vi "Timestamp_with_milliseconds.vi"(0 "Input Time":string="07:54:55.584 08/08/18") -> (4 "Output Time":string)   [LabVIEW 2014]
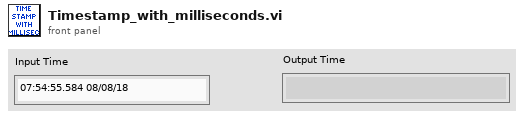
[diagram p1: front panel]
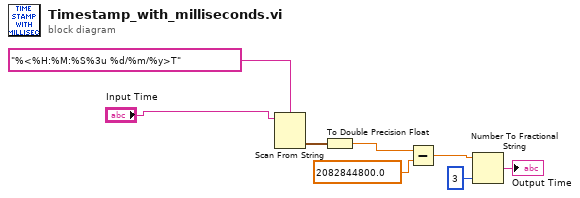
[diagram p0: block diagram]
diagram:
  n1 = Scan From String(format string="%<%H:%M:%S%3u %d/%m/%y>T", input string="Input Time") -> (output 1=w7:timestamp)  [unwired: 3 in, 3 out]
  n2 = To Double Precision Float(number=w7) -> (double precision float=w4:dbl)
  n3 = Subtract(x=w4, y=2082844800.0) -> (x-y=w3:dbl)
  n4 = Number To Fractional String(number=w3, precision (6)=i16 3) -> (F-format string=→"Output Time":string)  [unwired: 2 in]
